vi "correct angle.vi"(10 "Robot angle":dbl, 11 "Angle moved":dbl) -> (3 "Final angle":dbl)   [LabVIEW 2015]
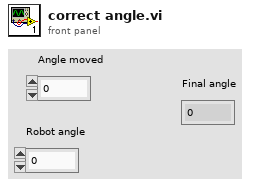
[diagram p1: front panel]
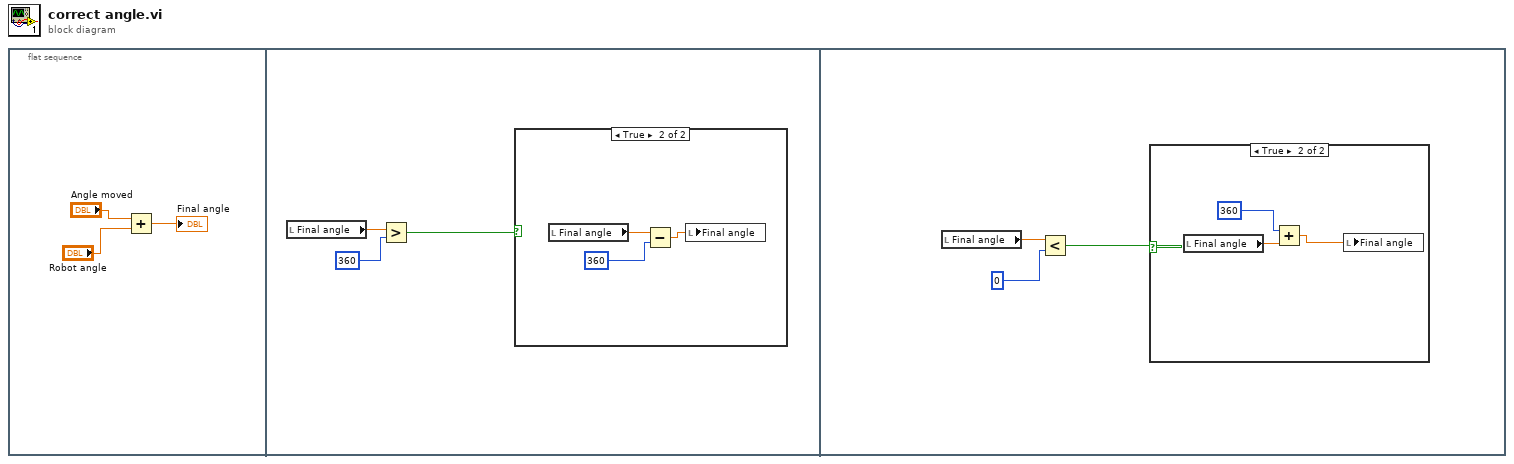
[diagram p0: block diagram]
diagram:
  n1 = flat-sequence {
    frame #0 {
      n2 = Add(x="Angle moved", y="Robot angle") -> (x+y=→"Final angle":dbl)
    }
    frame #1 {
      n3 = local read "Final angle"() -> (w6:dbl)
      n4 = Greater?(x=w6, y=360) -> (0:w4:bool)
      n5 = case shown="True" w4 {
        frame False {
        }
        frame True {
          n6 = local read "Final angle"() -> (w9:dbl)
          n7 = Subtract(x=w9, y=360) -> (x-y=w7:dbl)
          n8 = local write "Final angle"(w7) -> ()
        }
      }
    }
    frame #2 {
      n9 = local read "Final angle"() -> (w12:dbl)
      n10 = Less?(x=w12, y=0) -> (x < y?=w10:bool)
      n11 = case shown="True" w10 {
        frame False {
        }
        frame True {
          n12 = local read "Final angle"() -> (w15:dbl)
          n13 = Add(x=360, y=w15) -> (x+y=w13:dbl)
          n14 = local write "Final angle"(w13) -> ()
        }
      }
    }
  }
